vi "BLM_ReadOneNVmemory.vi"(4 "Read Echo?":bool, 5 "error in (no error)":errorcluster, 6 "Transit \nuser-defined register#":string, 7 "NV memory #":string, 8 "Port Address":refnum<visa-resource-name>) -> (0 "error out":errorcluster, 1 "NV memory value":dbl, 2 "NV memory string":string, 3 "Port Address Out":refnum<visa-resource-name>)   [LabVIEW 2021]
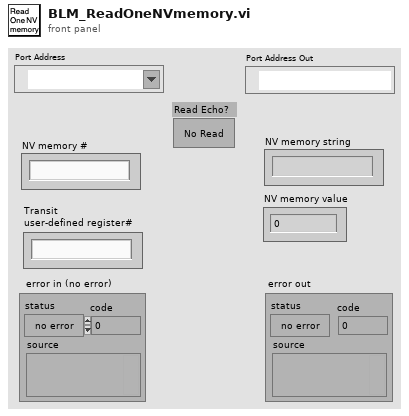
[diagram p1: front panel]
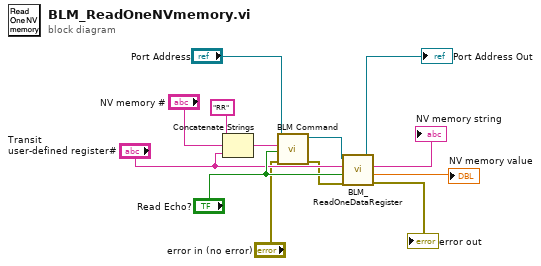
[diagram p0: block diagram]
diagram:
  n1 = Concatenate Strings("RR" ("string"), "NV memory #", "Transit \nuser-defined register#") -> (w10:string)
  n2 = call "BLM Command.vi"("error in (no error)"="error in (no error)", "Read Echo?"="Read Echo?", "Command"=w10, "Port Address"="Port Address") -> ("error out"=w3:errorcluster, "Port Address Out"=w4:refnum<visa-resource-name>)  [unwired: 2 in, 3 out]
  n3 = call "BLM_ReadOneDataRegister.vi"("error in (no error)"=w3, "Read Echo?"="Read Echo?", "Register#"="Transit \nuser-defined register#", "Port Address"=w4) -> ("error out"=→"error out":errorcluster, "Register Value"=→"NV memory value":dbl, "Register String"=→"NV memory string":string, "Port Address Out"=→"Port Address Out":refnum<visa-resource-name>)
